vi "heartbeat.vi"(8 "error in (no error)":errorcluster, 11 "MonoClientCommunicator in":refnum<class "MonoClientCommunicator.lvclass">) -> (0 "error out":errorcluster, 1 "newValue":bool, 2 "DeviceStatus":T1, 3 "MonoClientCommunicator out":refnum<class "MonoClientCommunicator.lvclass">)   [LabVIEW 2016, in "MonoClientCommunicator.lvclass"]
uses:
  MonoClientCommunicator.lvclass
  Typedefs/DeviceStatus.ctl
  MonoClientCommunicator.lvclass/MonoClientCommunicator.ctl
  MonoHeartbeat/MonoHeartbeat.lvclass
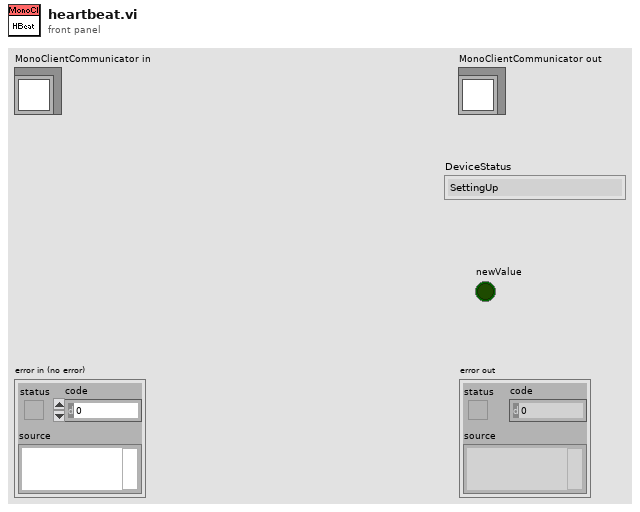
[diagram p1: front panel]
types:
  T1 = typedef "DeviceStatus.ctl" = enum16{"SettingUp", "Ready", "Offline", "Fault"}
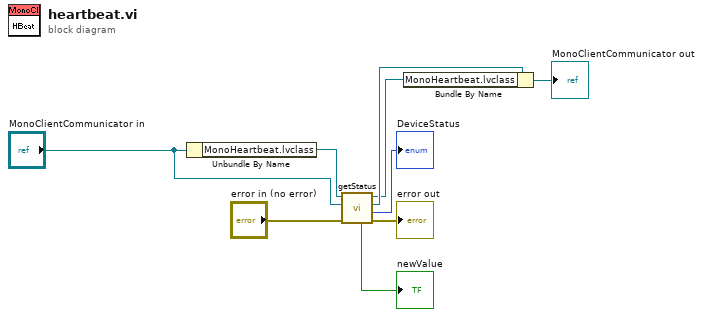
[diagram p0: block diagram]
diagram:
  n1 = Unbundle By Name("MonoClientCommunicator in") -> ("MonoHeartbeat.lvclass"=w9:refnum<class "MonoHeartbeat.lvclass">)
  n2 = call "getStatus.vi"("error in (no error)"="error in (no error)", "MonoClientCommunicator in"="MonoClientCommunicator in", "MonoHeartbeat in"=w9) -> ("error out"=→"error out":errorcluster, "DeviceStatus"=→"DeviceStatus":T1, "MonoClientCommunicator out"=w3:refnum<class "MonoClientCommunicator.lvclass">, "MonoHeartbeat out"=w1:refnum<class "MonoHeartbeat.lvclass">, "newValue"=→"newValue":bool)  [unwired: 4 in]
  n3 = Bundle By Name(cluster=w3, "MonoHeartbeat.lvclass"=w1) -> (→"MonoClientCommunicator out":refnum<class "MonoClientCommunicator.lvclass">)
